vi "Test Thermal Chamber API.vi"() -> ()   [LabVIEW 2024]
doc: "Thermal Chamber API Tester.\n\n<b>Note:</b> This VI was modified by the <b>Validate DQMH Module</b> tool to add the 'Show Main VI Diagram on Init' functionality included in DQMH 6.1.\n\n<b>Note:</b> This VI was modified by the <b>Validate DQMH Module</b> tool to upgrade its Error Reported event frame to use an improved mechanism for displaying error information.\n\n<b>Note:</b> This VI was modified by the <b>Validate DQMH Module</b> tool to remove code to stop the main loop on error, and instead display the most recent error on the tester front panel."
uses:
  Class Libraries/Process Controller/Controls/Temp Data--Cluster.ctl
  Class Libraries/Process Controller/Controls/Temperature Units--Enum.ctl
  Class Libraries/Process Controller/Controls/Temp Ramp Rate Data--Cluster.ctl
  Class Libraries/Process Controller/Controls/Rate Units--Enum.ctl
  Class Libraries/Process Controller/Controls/Class Selector--Enum.ctl
  <vilib>/Utility/error.llb/DialogType.ctl
  Thermal Chamber.lvlib
  <userlib>/_OpenG.lib/time/time.llb/openg_time.lvlib
  Class Libraries/Process Controller/_Thermal Process Controller.lvclass
panel:
  out "error out":errorcluster
  in  "Show Main VI Diagram on Init (F)":bool
  in  "File Path":path
  in  "Log Data?":bool
  in  "Class Types":T1
  in  "Temp Units":T2
  out "Temp Feedback":dbl
  in  "Temp Control State":bool
  in  "Temp Ramp Data":T3={"Temp Ramp Rate"=0.0, "Temp Units"=enum."Degrees C", "Rate Units"=enum."Degrees/Minutes"}
  in  "Temp Data":T5={"Temp"=0.0, "Temp Units"=enum."Degrees C"}
  in  "Get Temp Feedback":bool
  in  "Set Temp Control State":bool
  in  "Set Temp Ramp Rate":bool
  in  "Set Temp Setpoint":bool
  in  "Process Controller Shut Down":bool
  in  "VISA":refnum<visa-resource-name>
  in  "Initialize":bool
  in  "Run as Singleton?":bool
  in  "Show Block Diagram":bool
  in  "Refresh Modules":bool
  out "Active Modules":string[](array[string])
  in  "Stop Module":bool
  in  "Select Module":i32(ring)=-1 caption="Select Module\nTo send Request to" items=["All"=-1]
  in  "Run New Module":bool
  in  "Hide Module Panel":bool
  in  "Show Module Panel":bool
  out "Status":string
  # "This VI tests the API for the Module."
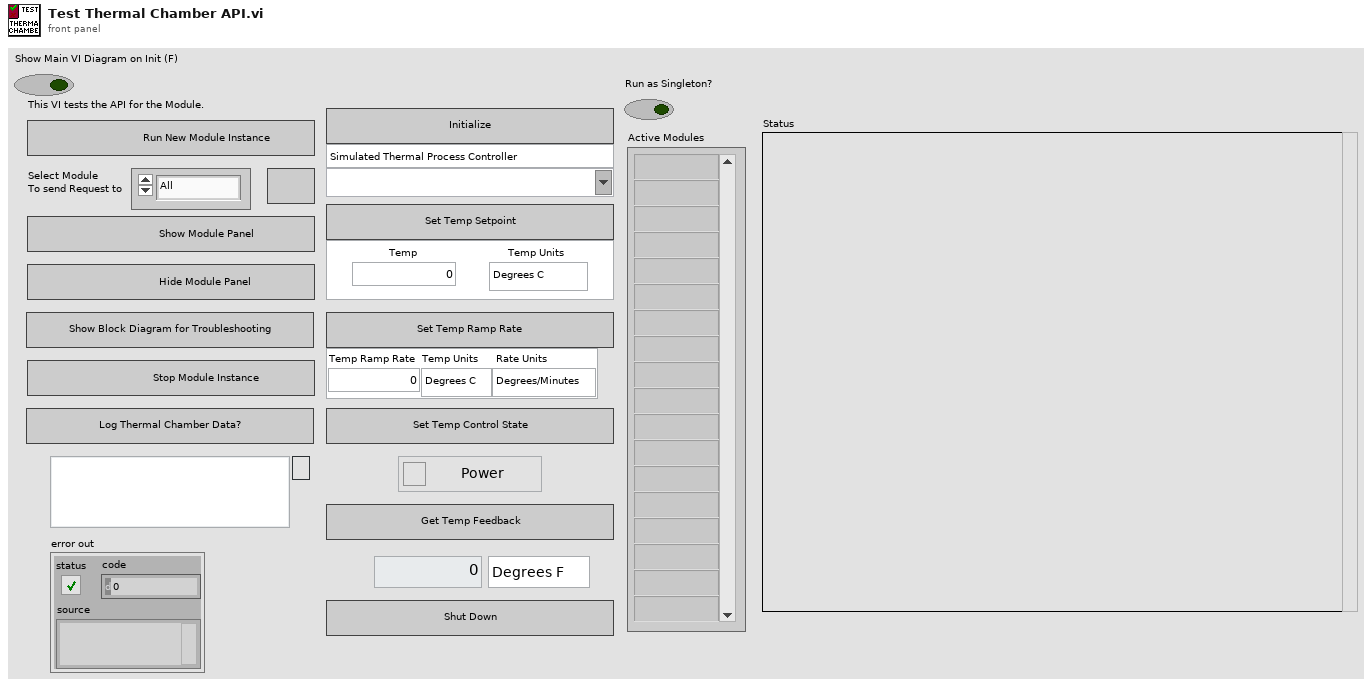
[diagram p1: front panel]
types:
  T1 = typedef "_Thermal Process Controller.lvclass/Class Selector--Enum.ctl" = enum16{"Simulated Thermal Process Controller", "Watlow F4T"}
  T2 = typedef "_Thermal Process Controller.lvclass/Temperature Units--Enum.ctl" = enum16{"Degrees F", "Degrees C", "Degrees K"}
  T3 = typedef "_Thermal Process Controller.lvclass/Temp Ramp Rate Data--Cluster.ctl" = cluster{"Temp Ramp Rate":dbl, "Temp Units":T2, "Rate Units":T4}
  T4 = typedef "_Thermal Process Controller.lvclass/Rate Units--Enum.ctl" = enum16{"Degrees/Minutes", "Degrees/Hours"}
  T5 = typedef "_Thermal Process Controller.lvclass/Temp Data--Cluster.ctl" = cluster{"Temp":dbl, "Temp Units":T2}
  T6 = cluster{"Stop":refnum<user-event>, "Logging":refnum<user-event>}
  T7 = typedef "Thermal Chamber.lvlib/Broadcast Events--cluster.ctl" = cluster{"Module Did Init":refnum<user-event>, "Status Updated":refnum<user-event>, "Error Reported":refnum<user-event>, "Module Did Stop":refnum<user-event>, "Update Module Execution Status":refnum<user-event>, "Ready":refnum<user-event>}
  T8 = typedef "DialogType.ctl" = u16
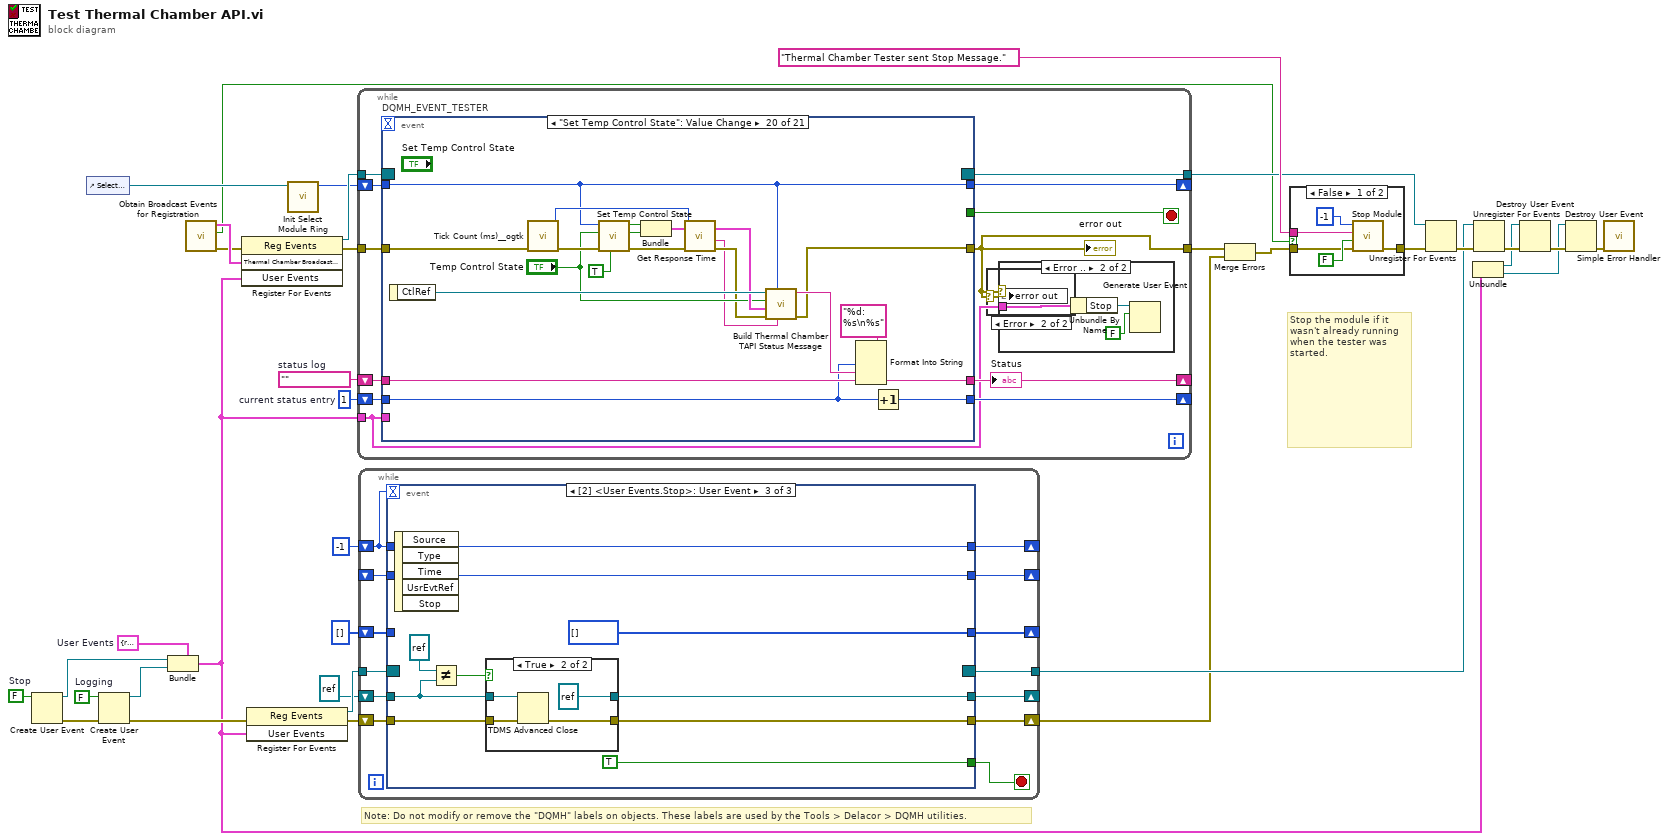
[diagram p0: block diagram]
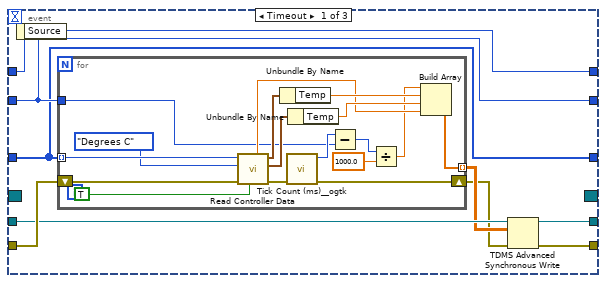
[diagram p2: hidden frame]
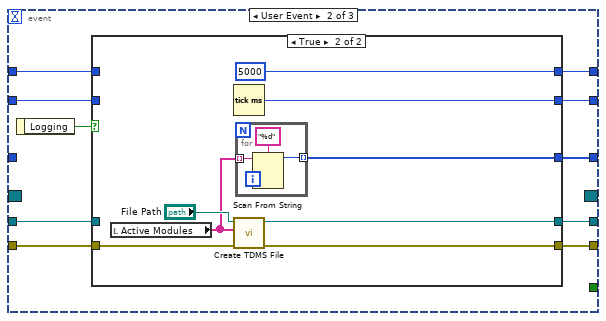
[diagram p3: hidden frame]
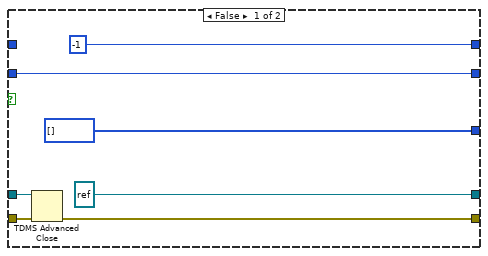
[diagram p4: hidden frame]
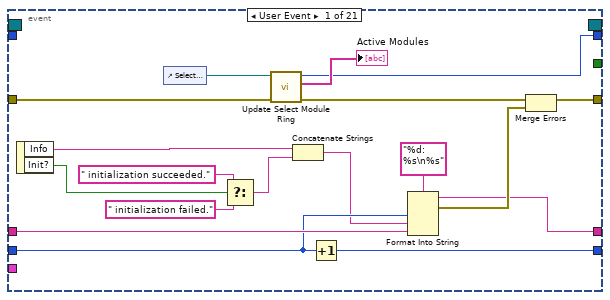
[diagram p9: hidden frame]
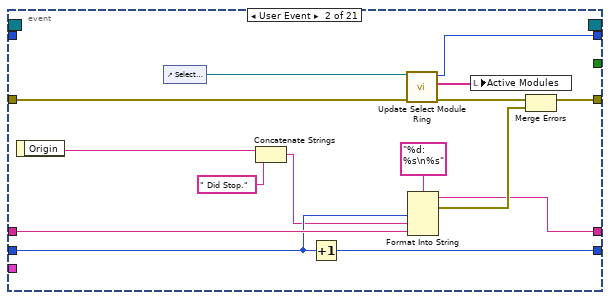
[diagram p10: hidden frame]
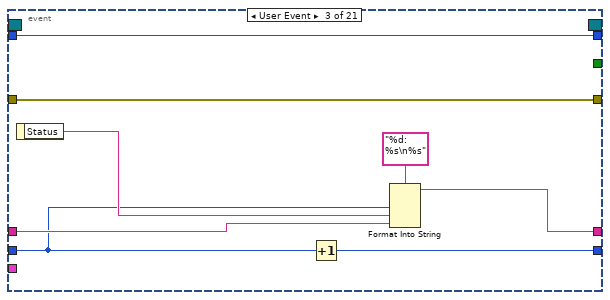
[diagram p11: hidden frame]
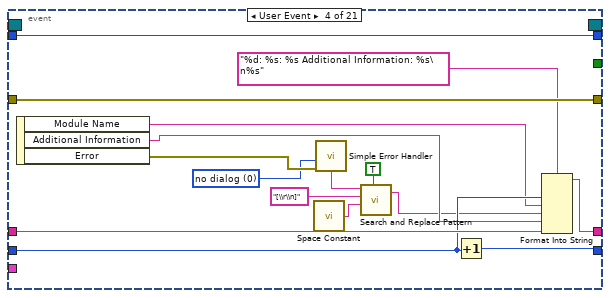
[diagram p12: hidden frame]
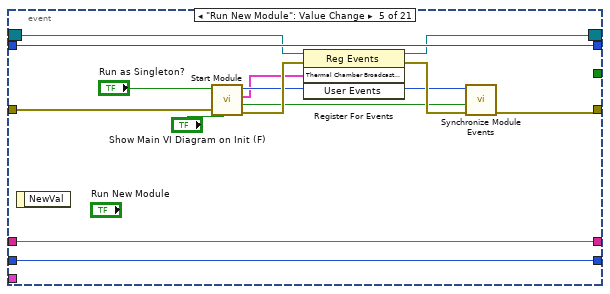
[diagram p13: hidden frame]
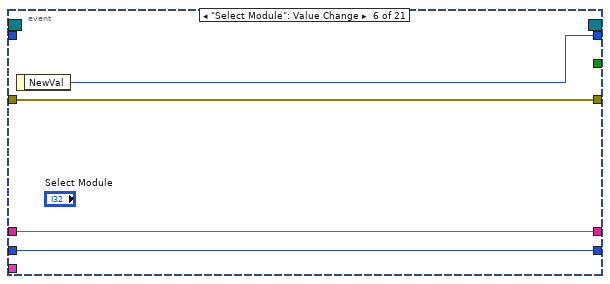
[diagram p14: hidden frame]
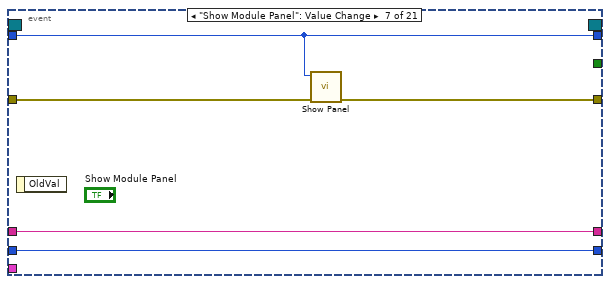
[diagram p15: hidden frame]
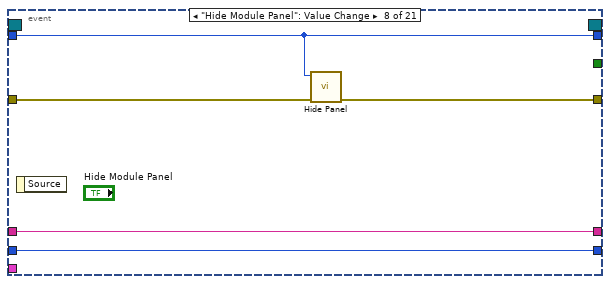
[diagram p16: hidden frame]
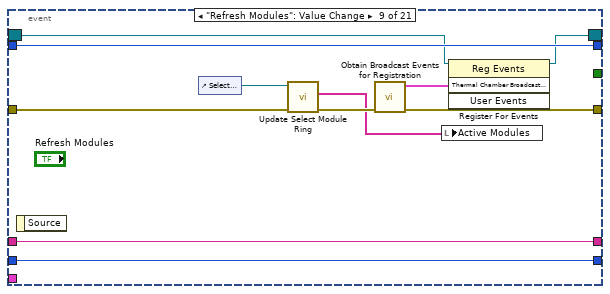
[diagram p17: hidden frame]
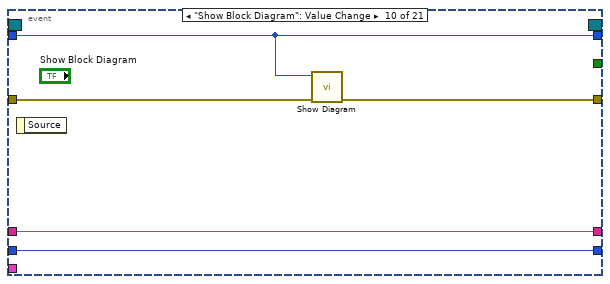
[diagram p18: hidden frame]
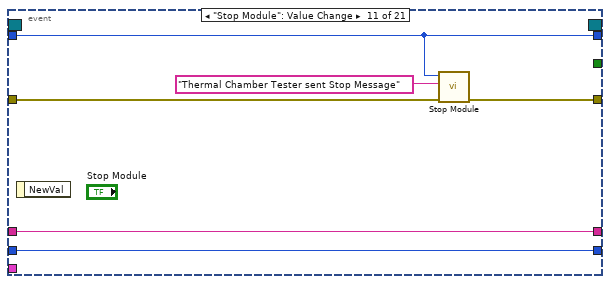
[diagram p19: hidden frame]
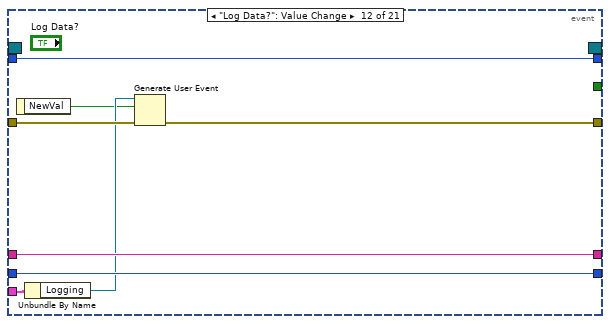
[diagram p20: hidden frame]
diagram:
  w8 = T6 {"Stop"=refnum, "Logging"=refnum}  # User Events
  w16 = FALSE  # Stop
  w23 = FALSE  # Logging
  w32 = 1  # current status entry
  w33 = ""  # status log
  # "Stop the module if it wasn't already running when the tester was started."
  # "Note: Do not modify or remove the \"DQMH\" labels on objects. These labels are used by the Tools > Delacor > DQMH utilities."
  n1 = Create User Event(user event datatype=w16) -> (user event=w12:refnum<user-event>, error out=w15:errorcluster)  [unwired: 1 in]
  n2 = control-ref of="Select Module"() -> (w30:refnum<vi>)
  n3 = Create User Event(user event datatype=w23, error in=w15) -> (user event=w13:refnum<user-event>, error out=w14:errorcluster)
  n4 = Bundle(cluster=w8, "Stop"=w12, "Logging"=w13) -> (w9:T6)
  n5 = call "Obtain Broadcast Events for Registration.vi"() -> ("error out"=w25:errorcluster, "Already running?"=w24:bool, "Thermal Chamber Broadcast Events"=w29:T7)  [unwired: 9 in]
  n6 = register-events(error in=w25, w29, w9) -> (reference out=w35:refnum<event-registration>, error out=w28:errorcluster)  [unwired: 1 in]
  n7 = register-events(error in=w14, w9) -> (reference out=w22:refnum<event-registration>, error out=w6:errorcluster)  [unwired: 1 in]
  n8 = call "Init Select Module Ring.vi"("Select Module Ring Ref"=w30) -> ("Value for All Modules"=w31:i32)  [unwired: 8 in, 2 out]
  n9 = while {
    tunnel: w35 -> [w47]
    tunnel: [w37] -> w3
    tunnel: w28 -> [w46]
    shift-right: [w42] -> _
    shift-left: w33 -> [w44]
    shift-right: [w43] -> _
    shift-left: w32 -> [w45]
    shift-right: [w39] -> _
    shift-left: w31 -> [w40]
    tunnel: [w38] -> w26
    tunnel: w9 -> [w36]
    stop <- w41 stop-if-true
    n10 = event "DQMH_EVENT_TESTER" shown="[19] \"Set Temp Control State\": Value Change" {
      selector: w47 -> [_ _ _ _ w116 _ _ _ w142 _ _ _ _ _ _ _ _ _ _ _ _]
      dyn-events: [_ _ _ _ w115 _ _ _ w141 _ _ _ _ _ _ _ _ _ _ _ _] -> w38
      timeout: _ -> [_ _ _ _ _ _ _ _ _ _ _ _ _ _ _ _ _ _ _ _ _]
      tunnel: [_ _ _ _ _ _ _ _ _ _ _ _ w175 _ _ _ _ _ _ _ _] -> w41
      tunnel: [w59 w76 w92 w107 w114 w126 w130 w135 w138 w149 w154 w162 w170 w178 w185 w215 w217 w237 w256 w278 w308] -> w37
      tunnel: w46 -> [w61 w78 w92 w107 w117 w126 w131 w136 w143 w152 w155 w163 w171 w179 w190 w215 w224 w243 w265 w288 w298]
      tunnel: w45 -> [w66 w81 w85 w104 w119 w124 w128 w133 w146 w150 w157 w165 w173 w181 w201 w206 w228 w246 w254 w277 w304]
      tunnel: w44 -> [w67 w82 w88 w106 w120 w125 w129 w134 w147 w151 w158 w166 w174 w182 w187 w213 w226 w248 w269 w281 w307]
      tunnel: [w64 w79 w89 w105 w120 w125 w129 w134 w147 w151 w158 w166 w174 w182 w200 w212 w225 w247 w268 w280 w306] -> w42
      tunnel: [w65 w80 w91 w103 w119 w124 w128 w133 w146 w150 w157 w165 w173 w181 w202 w211 w227 w245 w253 w276 w303] -> w43
      tunnel: w40 -> [_ _ w86 w108 w118 _ w127 w132 w145 w148 w156 w164 w172 _ w199 w214 w219 w238 w257 w274 w294]
      tunnel: [w56 w73 w86 w108 w118 w123 w127 w132 w145 w148 w156 w164 w172 w177 w199 w214 w219 w238 w257 w274 w294] -> w39
      tunnel: w36 -> [_ _ _ _ _ _ _ _ _ _ _ w161 w169 _ _ _ _ _ _ _ _]
      event User Event {
        n11 = event-data() -> ("Info"=w63:string, "Init?"=w53:bool)  [unwired: 1 in]
        n12 = control-ref of="Select Module"() -> (w58:refnum<vi>)
        n13 = Select(t=" initialization succeeded.", s=w53, f=" initialization failed.") -> (s? t:f=w52:string)
        n14 = call "Update Select Module Ring.vi"("error in (no error)"=w61, "Select Module Ring Ref"=w58) -> ("error out"=w60:errorcluster, "Active Modules (Array)"=→"Active Modules":string[], "New Module Ring Value"=w56:i32)  [unwired: 7 in]
        n15 = Concatenate Strings(w63, w52) -> (w62:string)
        n16 = Increment(x=w66) -> (x+1=w65:i32)
        n17 = Format Into String(format string="%d: %s\n%s", w66, w62, w67) -> (resulting string=w64:string, error out=w69:errorcluster)  [unwired: 2 in]
        n18 = Merge Errors(w60, w69) -> (w59:errorcluster)
      }
      event User Event {
        n19 = event-data() -> ("Origin"=w71:string)  [unwired: 1 in]
        n20 = control-ref of="Select Module"() -> (w75:refnum<vi>)
        n21 = Concatenate Strings(w71, " Did Stop.") -> (w70:string)
        n22 = Increment(x=w81) -> (x+1=w80:i32)
        n23 = call "Update Select Module Ring.vi"("error in (no error)"=w78, "Select Module Ring Ref"=w75) -> ("error out"=w77:errorcluster, "Active Modules (Array)"=w74:string[], "New Module Ring Value"=w73:i32)  [unwired: 7 in]
        n24 = Format Into String(format string="%d: %s\n%s", w81, w70, w82) -> (resulting string=w79:string, error out=w84:errorcluster)  [unwired: 2 in]
        n25 = local write "Active Modules"(w74) -> ()
        n26 = Merge Errors(w77, w84) -> (w76:errorcluster)
      }
      event User Event {
        n27 = event-data() -> ("Status"=w87:string)  [unwired: 1 in]
        n28 = Increment(x=w85) -> (x+1=w91:i32)
        n29 = Format Into String(format string="%d: %s\n%s", w85, w87, w88) -> (resulting string=w89:string)  [unwired: 2 in, 1 out]
      }
      event User Event {
        w99 = T8 0 items=["no dialog", "OK message", "continue or stop message", "OK message + warnings", "continue/stop + warnings"] ("type of dialog (OK msg:1)")
        n30 = event-data() -> ("Module Name"=w100:string, "Additional Information"=w101:string, "Error"=w102:errorcluster)  [unwired: 1 in]
        n31 = call <vilib>:"Space Constant.vi"() -> ("String"=w95:string)
        n32 = call <vilib>:"Simple Error Handler.vi"("type of dialog (OK msg:1)"=w99, "error in (no error)"=w102) -> ("message"=w98:string)  [unwired: 3 in, 4 out]
        n33 = call <vilib>:"Search and Replace Pattern.vi"("string"=w98, "regular expression (\"\")"="[\\r\\n]" ("regular expression (\"\")"), "replace string (\"\")"=w95, "replace all? (F)"=TRUE ("replace all CR/LF with spaces")) -> ("result string"=w97:string)  [unwired: 1 in, 1 out]
        n34 = Increment(x=w104) -> (x+1=w103:i32)
        n35 = Format Into String(format string="%d: %s: %s Additional Information: %s\n%s", w104, w100, w97, w101, w106) -> (resulting string=w105:string)  [unwired: 2 in, 1 out]
      }
      event "Run New Module": Value Change {
        n36 = event-data() -> ()  [unwired: 1 in, 1 out]
        n37 = call "Start Module.vi"("Show Main VI Diagram on Init (F)"="Show Main VI Diagram on Init (F)", "error in"=w117, "Run as Singleton? (F)"="Run as Singleton?") -> ("error out"=w121:errorcluster, "Wait for Event Sync?"=w112:bool, "Thermal Chamber Broadcast Events"=w111:T7, "Module ID"=w113:i32)  [unwired: 5 in]
        n38 = register-events(reference=w116, error in=w121, w111) -> (reference out=w115:refnum<event-registration>, error out=w122:errorcluster)  [unwired: 1 in]
        n39 = call "Synchronize Module Events.vi"("error in"=w122, "Wait for Event Sync?"=w112, "Module ID in"=w113) -> ("error out"=w114:errorcluster)  [unwired: 7 in, 1 out]
      }
      event "Select Module": Value Change {
        n40 = event-data() -> ("NewVal"=w123:i32)  [unwired: 1 in]
      }
      event "Show Module Panel": Value Change {
        n41 = event-data() -> ()  [unwired: 1 in, 1 out]
        n42 = call "Show Panel.vi"("error in (no error)"=w131, "Module ID"=w127) -> ("error out"=w130:errorcluster)  [unwired: 9 in]
      }
      event "Hide Module Panel": Value Change {
        n43 = event-data() -> ()  [unwired: 1 in, 1 out]
        n44 = call "Hide Panel.vi"("error in (no error)"=w136, "Module ID"=w132) -> ("error out"=w135:errorcluster)  [unwired: 9 in]
      }
      event "Refresh Modules": Value Change {
        n45 = event-data() -> ()  [unwired: 1 in, 1 out]
        n46 = control-ref of="Select Module"() -> (w144:refnum<vi>)
        n47 = call "Update Select Module Ring.vi"("error in (no error)"=w143, "Select Module Ring Ref"=w144) -> ("error out"=w139:errorcluster, "Active Modules (Array)"=w137:string[])  [unwired: 7 in, 1 out]
        n48 = call "Obtain Broadcast Events for Registration.vi"("error in (no error)"=w139) -> ("error out"=w138:errorcluster, "Thermal Chamber Broadcast Events"=w140:T7)  [unwired: 8 in, 1 out]
        n49 = local write "Active Modules"(w137) -> ()
        n50 = register-events(reference=w142, w140) -> (reference out=w141:refnum<event-registration>)  [unwired: 2 in, 1 out]
      }
      event "Show Block Diagram": Value Change {
        n51 = event-data() -> ()  [unwired: 1 in, 1 out]
        n52 = call "Show Diagram.vi"("error in (no error)"=w152, "Module ID"=w148) -> ("error out"=w149:errorcluster)  [unwired: 9 in]
      }
      event "Stop Module": Value Change {
        n53 = event-data() -> ()  [unwired: 1 in, 1 out]
        n54 = call "Stop Module.vi"("error in (no error)"=w155, "Origin"="Thermal Chamber Tester sent Stop Message", "Module ID"=w156) -> ("error out"=w154:errorcluster)  [unwired: 8 in]
      }
      event "Log Data?": Value Change {
        n55 = event-data() -> ("NewVal"=w159:bool)  [unwired: 1 in]
        n56 = Unbundle By Name(w161) -> ("Logging"=w160:refnum<user-event>)
        n57 = Generate User Event(user event=w160, event data cluster=w159, error in=w163) -> (error out=w162:errorcluster)  [unwired: 1 in, 1 out]
      }
      event Panel Close? {
        w175 = TRUE ("Discard?")
        n58 = event-data() -> ()  [unwired: 1 in, 1 out]
        n59 = Unbundle By Name(w169) -> ("Stop"=w168:refnum<user-event>)
        n60 = Generate User Event(user event=w168, event data cluster=FALSE ("event data"), error in=w171) -> (error out=w170:errorcluster)  [unwired: 1 in, 1 out]
        n61 = event-data("Discard?"=w175) -> ()  [unwired: 1 in, 1 out]
      }
      event User Event {
        # "Update the active modules list whenever the module execution status is updated. Note that this event should only ever fire when Start Module VI is called for a cloneable running as singleton, but the module is already running."
        n62 = event-data() -> ()  [unwired: 1 in, 1 out]
        n63 = control-ref of="Select Module"() -> (w180:refnum<vi>)
        n64 = call "Update Select Module Ring.vi"("error in (no error)"=w179, "Select Module Ring Ref"=w180) -> ("error out"=w178:errorcluster, "Active Modules (Array)"=w176:string[], "New Module Ring Value"=w177:i32)  [unwired: 7 in]
        n65 = local write "Active Modules"(w176) -> ()
      }
      event "Initialize": Value Change {
        w203 = TRUE  # wait for reply (T)
        n66 = event-data() -> ()  [unwired: 1 in, 1 out]
        n67 = call <userlib>:"Tick Count (ms)__ogtk.vi"("error in (no error)"=w190) -> ("error out"=w189:errorcluster, "millisecond timer value"=w186:u32)  [unwired: 9 in]
        n68 = call "Initialize.vi"("wait for reply (T)"=w203, "error in"=w189, "VISA"="VISA", "Class Types"="Class Types", "Module ID"=w199) -> ("error out"=w188:errorcluster, "Ready"=w197:bool)  [unwired: 4 in, 1 out]
        n69 = Boolean To (0,1)(Boolean=w197) -> (0, 1=w198:i16)
        n70 = To Long Integer(number=w198) -> (32bit integer=w183:i32)
        n71 = call "Get Response Time.vi"("error in (no error)"=w188, "Start Count"=w186) -> ("error out"=w185:errorcluster, "Response Time String"=w184:string)  [unwired: 8 in]
        n72 = Pick Line(string ("")="Attempting to Connect to Controller...." ("format string"), multi-line string="Connection Failed\nConnection Successful" ("string (\"\")"), line index=w183) -> (output string=w193:string)
        n73 = Increment(x=w201) -> (x+1=w202:i32)
        n74 = Format Into String(format string="%d: Chamber(%d) %s... %s\n%s", w201, w199, w193, w184, w187) -> (resulting string=w200:string)  [unwired: 2 in, 1 out]
      }
      event User Event {
        # "Why?"
        n75 = event-data() -> ("Module ID"=w204:i32, "Ready"=w207:bool)  [unwired: 1 in]
        n76 = Select(t="Ready" ("format string"), s=w207, f="Not Ready") -> (s? t:f=w205:string)
        n77 = Increment(x=w206) -> (x+1=w211:i32)
        n78 = Format Into String(format string="%d: Response Received - Thermal Chamber(%d) %s\n%s", w206, w204, w205, w213) -> (resulting string=w212:string)  [unwired: 2 in, 1 out]
      }
      event "Process Controller Shut Down": Value Change {
        n79 = event-data() -> ()  [unwired: 1 in, 1 out]
        n80 = call <userlib>:"Tick Count (ms)__ogtk.vi"("error in (no error)"=w224) -> ("error out"=w223:errorcluster, "millisecond timer value"=w221:u32)  [unwired: 9 in]
        n81 = call "Shutdown.vi"("wait for reply (T)"=TRUE, "error in"=w223, "Module ID in"=w219) -> ("error out"=w222:errorcluster)  [unwired: 5 in, 3 out]
        n82 = call "Get Response Time.vi"("error in (no error)"=w222, "Start Count"=w221) -> ("error out"=w217:errorcluster, "Response Time String"=w216:string)  [unwired: 8 in]
        n83 = Format Into String(format string="Request Shut Down Process Controller(%d)---%s", w219, w216) -> (resulting string=w218:string)  [unwired: 2 in, 1 out]
        n84 = Increment(x=w228) -> (x+1=w227:i32)
        n85 = Format Into String(format string="%d: %s\n%s", w228, w218, w226) -> (resulting string=w225:string)  [unwired: 2 in, 1 out]
      }
      event "Set Temp Setpoint": Value Change {
        n86 = event-data() -> ("CtlRef"=w240:refnum<vi>)  [unwired: 1 in]
        n87 = call <userlib>:"Tick Count (ms)__ogtk.vi"("error in (no error)"=w243) -> ("error out"=w242:errorcluster, "millisecond timer value"=w241:u32)  [unwired: 9 in]
        n88 = call "Set Temp Setpoint.vi"("wait for reply (T)"=TRUE, "error in"=w242, "Temp Setpoint Data in"="Temp Data", "Module ID"=w238) -> ("error out"=w244:errorcluster, "Temp Setpoint Data"=w234:T5, "Set?"=w235:bool)  [unwired: 4 in, 1 out]
        n89 = Bundle("Set?"=w235, "Temp Setpoint Data"=w234) -> (w233:cluster{"Set?":bool, "Temp Setpoint Data":T5})  [unwired: 1 in]
        n90 = call "Get Response Time.vi"("error in (no error)"=w244, "Start Count"=w241) -> ("error out"=w232:errorcluster, "Response Time String"=w231:string)  [unwired: 8 in]
        n91 = call "Build Thermal Chamber TAPI Status Message.vi"("Response Time"=w231, "Module ID"=w238, "error in"=w232, "Reply Data"=w233, "Request/Broadcast Data"="Temp Data", "CtlRef"=w240) -> ("error out"=w237:errorcluster, "Message"=w236:string)  [unwired: 4 in]
        n92 = Increment(x=w246) -> (x+1=w245:i32)
        n93 = Format Into String(format string="%d: %s\n%s", w246, w236, w248) -> (resulting string=w247:string)  [unwired: 2 in, 1 out]
      }
      event "Set Temp Ramp Rate": Value Change {
        (unwired) T3 {"Temp Ramp Rate"=5.0, "Temp Units"=enum."Degrees F", "Rate Units"=enum."Degrees/Minutes"} ("Temp Ramp Data")
        (unwired) cluster{"Set?":bool, "Temp Ramp Data":T3} {"Set?"=FALSE, "Temp Ramp Data"={"Temp Ramp Rate"=0.0, "Temp Units"=enum."Degrees F", "Rate Units"=enum."Degrees/Minutes"}} ("output cluster")
        n94 = event-data() -> ("CtlRef"=w259:refnum<vi>)  [unwired: 1 in]
        n95 = call <userlib>:"Tick Count (ms)__ogtk.vi"("error in (no error)"=w265) -> ("error out"=w264:errorcluster, "millisecond timer value"=w261:u32)  [unwired: 9 in]
        n96 = call "Set Temp Ramp Rate.vi"("wait for reply (T)"=TRUE, "error in"=w264, "Temp Ramp Data in"="Temp Ramp Data", "Module ID"=w257) -> ("error out"=w262:errorcluster, "Temp Ramp Data"=w266:T3, "Set?"=w267:bool)  [unwired: 4 in, 1 out]
        n97 = Bundle("Set?"=w267, "Temp Ramp Data"=w266) -> (w258:cluster{"Set?":bool, "Temp Ramp Data":T3})  [unwired: 1 in]
        n98 = call "Get Response Time.vi"("error in (no error)"=w262, "Start Count"=w261) -> ("error out"=w252:errorcluster, "Response Time String"=w251:string)  [unwired: 8 in]
        n99 = call "Build Thermal Chamber TAPI Status Message.vi"("Response Time"=w251, "Module ID"=w257, "error in"=w252, "Reply Data"=w258, "Request/Broadcast Data"="Temp Ramp Data", "CtlRef"=w259) -> ("error out"=w256:errorcluster, "Message"=w255:string)  [unwired: 4 in]
        n100 = Format Into String(format string="%d: %s\n%s", w254, w255, w269) -> (resulting string=w268:string)  [unwired: 2 in, 1 out]
        n101 = Increment(x=w254) -> (x+1=w253:i32)
      }
      event "Set Temp Control State": Value Change {
        n102 = event-data() -> ("CtlRef"=w284:refnum<vi>)  [unwired: 1 in]
        n103 = call <userlib>:"Tick Count (ms)__ogtk.vi"("error in (no error)"=w288) -> ("error out"=w287:errorcluster, "millisecond timer value"=w285:u32)  [unwired: 9 in]
        n104 = call "Set Temp Control State.vi"("wait for reply (T)"=TRUE, "error in"=w287, "State in"="Temp Control State", "Module ID"=w274) -> ("error out"=w286:errorcluster, "State"=w290:bool, "Set?"=w289:bool)  [unwired: 4 in, 1 out]
        n105 = Bundle("Set?"=w289, "State"=w290) -> (w283:cluster{"Set?":bool, "State":bool})  [unwired: 1 in]
        n106 = call "Get Response Time.vi"("error in (no error)"=w286, "Start Count"=w285) -> ("error out"=w272:errorcluster, "Response Time String"=w271:string)  [unwired: 8 in]
        n107 = call "Build Thermal Chamber TAPI Status Message.vi"("Response Time"=w271, "Module ID"=w274, "error in"=w272, "Reply Data"=w283, "Request/Broadcast Data"="Temp Control State", "CtlRef"=w284) -> ("error out"=w278:errorcluster, "Message"=w279:string)  [unwired: 4 in]
        n108 = Format Into String(format string="%d: %s\n%s", w277, w279, w281) -> (resulting string=w280:string)  [unwired: 2 in, 1 out]
        n109 = Increment(x=w277) -> (x+1=w276:i32)
      }
      event "Get Temp Feedback": Value Change {
        n110 = event-data() -> ("CtlRef"=w299:refnum<vi>)  [unwired: 1 in]
        n111 = call <userlib>:"Tick Count (ms)__ogtk.vi"("error in (no error)"=w298) -> ("error out"=w297:errorcluster, "millisecond timer value"=w295:u32)  [unwired: 9 in]
        n112 = call "Get Temp Feedback.vi"("wait for reply (T)"=TRUE, "error in"=w297, "Temp Units"="Temp Units", "Module ID"=w294) -> ("error out"=w296:errorcluster, "Temp Feedback Data"=w301:T5)  [unwired: 5 in, 1 out]
        n113 = call "Get Response Time.vi"("error in (no error)"=w296, "Start Count"=w295) -> ("error out"=w291:errorcluster, "Response Time String"=w292:string)  [unwired: 8 in]
        n114 = Unbundle By Name(w301) -> ("Temp"=→"Temp Feedback":dbl)
        n115 = call "Build Thermal Chamber TAPI Status Message.vi"("Response Time"=w292, "Module ID"=w294, "error in"=w291, "Reply Data"=w301, "Request/Broadcast Data"="Temp Units", "CtlRef"=w299) -> ("error out"=w308:errorcluster, "Message"=w302:string)  [unwired: 4 in]
        n116 = Increment(x=w304) -> (x+1=w303:i32)
        n117 = Format Into String(format string="%d: %s\n%s", w304, w302, w307) -> (resulting string=w306:string)  [unwired: 2 in, 1 out]
      }
    }
    "Status" <- w42
    "error out" <- w37
    n118 = case "DQMH_TESTER_ERROR_LOCAL" shown="Error" w37 {
      selector: w37 -> [_ w48]
      frame No Error {
      }
      frame Error {
        n119 = local write "error out"(w48) -> ()
      }
    }
    n120 = case shown="Error .." w37 {
      tunnel: w36 -> [_ w49]
      frame No Error {
      }
      frame Error {
        n121 = Unbundle By Name(w49) -> ("Stop"=w50:refnum<user-event>)
        n122 = Generate User Event(user event=w50, event data cluster=FALSE ("event data")) -> ()  [unwired: 2 in, 2 out]
      }
    }
  }
  n123 = while {
    tunnel: w22 -> [w322]
    tunnel: [w321] -> w20
    shift-right: [w318] -> _
    shift-left: -1 -> [w319]
    shift-right: [w316] -> w1
    shift-left: w6 -> [w317]
    shift-right: [w315] -> _
    shift-left: refnum<k34> refnum ("tdms file out") -> [w314]
    shift-right: [w313] -> _
    shift-left: i32[] [] -> [w312]
    shift-right: [w311] -> _
    shift-left: _ -> [w310]
    stop <- w320 stop-if-true
    n124 = event shown="[2] <User Events.Stop>: User Event" {
      selector: w322 -> [_ _ _]
      dyn-events: [_ _ _] -> w321
      timeout: w319 -> [_ _ _]
      tunnel: [_ _ TRUE] -> w320
      tunnel: w319 -> [w331 w358 w385]
      tunnel: [w331 w357 w385] -> w318
      tunnel: w317 -> [w330 w355 w381]
      tunnel: [w326 w354 w380] -> w316
      tunnel: [w327 w353 w379] -> w315
      tunnel: w314 -> [w325 w352 w383]
      tunnel: [w328 w351 i32[] []] -> w313
      tunnel: w312 -> [w328 _ _]
      tunnel: [w329 w350 w377] -> w311
      tunnel: w310 -> [w329 w349 w377]
      event Timeout {
        n125 = event-data() -> ()  [unwired: 1 in, 1 out]
        n126 = for {
          tunnel: w328 -> [w348] mode=indexing
          shift-right: [w333] -> w323
          shift-left: w330 -> [w347]
          tunnel: [w339] -> w324 mode=indexing
          tunnel: w329 -> [w336]
          n127 = call "Read Controller Data.vi"("wait for reply (T)"=TRUE, "error in"=w347, "Temp Units"=Temperature_Units--Enum."Degrees C", "Module ID"=w348) -> ("error out"=w338:errorcluster, "Temp Setpoint"=w343:T5, "Chamber Temp"=w344:T5, "Chamber Output"=w340:dbl)  [unwired: 3 in, 1 out]
          n128 = Unbundle By Name(w344) -> ("Temp"=w342:dbl)
          n129 = call <userlib>:"Tick Count (ms)__ogtk.vi"("error in (no error)"=w338) -> ("error out"=w333:errorcluster, "millisecond timer value"=w337:u32)  [unwired: 9 in]
          n130 = Unbundle By Name(w343) -> ("Temp"=w341:dbl)
          n131 = Subtract(x=w337, y=w336) -> (x-y=w334:u32)
          n132 = Divide(x=w334, y=1000.0) -> (x/y=w332:dbl)
          n133 = Build Array(w332, w342, w341, w340) -> (w339:dbl[])
        }
        n134 = TDMS Advanced Synchronous Write(8:w323, 10:w324, 11:w325) -> (0:w326:errorcluster, 3:w327:refnum<k34>)
      }
      event User Event {
        n135 = event-data() -> ("Logging"=w356:bool)  [unwired: 1 in]
        n136 = case shown="True" w356 {
          tunnel: w358 -> [_ _]
          tunnel: [-1 5000] -> w357
          tunnel: w355 -> [w363 w371]
          tunnel: [w362 w370] -> w354
          tunnel: [refnum<k34> refnum ("tdms file out") w369] -> w353
          tunnel: w352 -> [w364 _]
          tunnel: [i32[] [] w367] -> w351
          tunnel: [w359 w366] -> w350
          tunnel: w349 -> [w359 _]
          frame False {
            n137 = TDMS Advanced Close(8:w363, 11:w364) -> (0:w362:errorcluster)  [unwired: 2 in, 1 out]
          }
          frame True {
            n138 = local read "Active Modules"() -> (w368:string[])
            n139 = Tick Count (ms)() -> (millisecond timer value=w366:u32)
            n140 = call "Create TDMS File.vi"("error in"=w371, "Active Modules"=w368, "file path"="File Path") -> ("error out"=w370:errorcluster, "tdms file out"=w369:refnum<k34>)  [unwired: 7 in]
            n141 = for {
              tunnel: w368 -> [w375] mode=indexing
              tunnel: [w374] -> w367 mode=indexing
              n142 = Scan From String(format string="%d", input string=w375) -> (output 1=w374:i32)  [unwired: 3 in, 3 out]
            }
          }
        }
      }
      event User Event {
        n143 = event-data() -> ()  [unwired: 1 in, 5 out]
        n144 = Not Equal?(x=refnum<k34> refnum ("tdms file out"), y=w383) -> (x != y?=w382:bool)
        n145 = case shown="True" w382 {
          tunnel: w383 -> [w388 w392]
          tunnel: w381 -> [w387 w391]
          tunnel: [w387 w390] -> w380
          tunnel: [w388 refnum<k34> refnum ("tdms file out")] -> w379
          frame False {
          }
          frame True {
            n146 = TDMS Advanced Close(8:w391, 11:w392) -> (0:w390:errorcluster)  [unwired: 2 in, 1 out]
          }
        }
      }
    }
  }
  n147 = Merge Errors(w3, w1) -> (w2:errorcluster)
  n148 = case shown="False" w24 {
    tunnel: [w397 w398] -> w34
    tunnel: "Thermal Chamber Tester sent Stop Message." ("Origin") -> [w396 _]
    tunnel: w2 -> [w393 w398]
    frame False {
      n149 = call "Stop Module.vi"("error in (no error)"=w393, "Wait for Module to stop? (F)"=FALSE ("Wait for Module to stop?"), "Origin"=w396, "Module ID"=-1 ("Stop all")) -> ("error out"=w397:errorcluster)  [unwired: 7 in]
    }
    frame True {
    }
  }
  n150 = Unregister For Events(event registration refnum=w26, error in=w34) -> (error out=w21:errorcluster)
  n151 = Unbundle(w9) -> ("Stop"=w11:refnum<user-event>, "Logging"=w10:refnum<user-event>)
  n152 = Unregister For Events(event registration refnum=w20, error in=w21) -> (error out=w19:errorcluster)
  n153 = Destroy User Event(user event=w11, error in=w19) -> (error out=w18:errorcluster)
  n154 = Destroy User Event(user event=w10, error in=w18) -> (error out=w17:errorcluster)
  n155 = call <vilib>:"Simple Error Handler.vi"("error in (no error)"=w17) -> ()  [unwired: 4 in, 5 out]
